vi "Is_ExtensionEXE.vi"(0 "path":path) -> (1 "Extension":string, 2 "Boolean":bool)   [LabVIEW 2011]
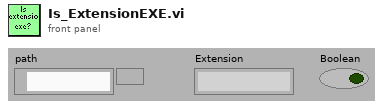
[diagram p1: front panel]
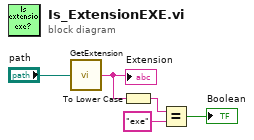
[diagram p0: block diagram]
diagram:
  n1 = call "GetExtension.vi"("path"="path") -> ("Extension"=w2:string)
  "Extension" <- w2
  n2 = To Lower Case(string=w2) -> (all lower case string=w3:string)
  n3 = Equal?(x=w3, y="exe") -> (x = y?=→"Boolean":bool)
